vi "Configure Null.vi"(8 "error in (no error)":errorcluster, 11 "34410A in":refnum<class "34410A.lvclass">) -> (0 "error out":errorcluster, 3 "34410A out":refnum<class "34410A.lvclass">)   [LabVIEW 2015, in "34410A.lvclass"]
uses:
  34410A.lvclass
  <instrlib>/Agilent 34401/Agilent 34401.lvlib
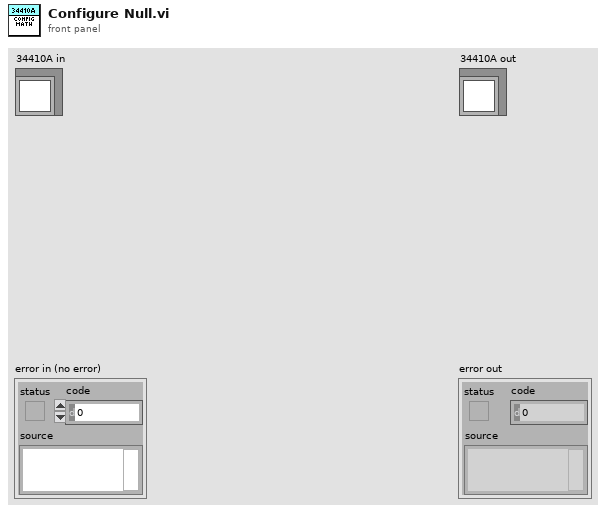
[diagram p1: front panel]
types:
  T1 = enum16{"None", "Min/Max", "Null", "dB", "dBm", "Limit"}
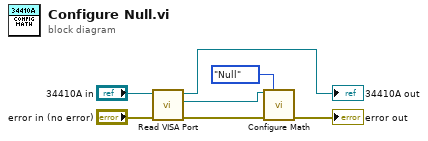
[diagram p0: block diagram]
diagram:
  n1 = call-dynamic "Read VISA Port.vi"("error in (no error)"="error in (no error)", "Device in"="34410A in") -> ("error out"=w1:errorcluster, "VISA Port"=w3:refnum<visa-resource-name>, "Device out"=→"34410A out":refnum<class "34410A.lvclass">)  [unwired: 7 in]
  n2 = call <instrlib>:"Configure Math.vi"("VISA resource name"=w3, "Operation (0:None)"=T1."Null", "error in (no error)"=w1) -> ("error out"=→"error out":errorcluster)  [unwired: 11 in, 1 out]
